vi "DAQ Frequency Meter.vi"() -> ()   [LabVIEW 2013]
doc: "Use this template to build a standard state machine design pattern. Each state executes code and determines which state to transition to. Contrast this design pattern with the User Interface Event Handler pattern, in which code executes in response to user actions. Contrast this design pattern also with the Queued Message Handler pattern, in which each message handling code can queue zero or more new messages.\nNote: This template does not contain the most recent programming guidelines recommended by National Instruments. For a complete, project-based implementation of the Standard State Machine pattern, use the Create Project dialog box instead of this template."
uses:
  DAQ_Count_States.ctl
  <vilib>/DAQmx/read.llb/DAQmx Read (Counter DBL 1Chan 1Samp).vi
  globals_9.vi
  <vilib>/DAQmx/create/channels.llb/DAQmx Create Channel (CI-Period).vi
  <vilib>/DAQmx/create/channels.llb/DAQmx Create Channel (CI-Frequency).vi
  <vilib>/DAQmx/miscellaneous.llb/DAQmx Fill In Error Info.vi
  <resource>/objmgr/daqmx.rc
panel:
  in  "stop":bool
  out "data":dbl caption="Frequency, Hz" format="%_8p"
  in  "mode":enum16{"period", "frequency"}(ring)
  in  "terminal":tag
  in  "counter":tag
  in  "measurement method":i32(ring)=10105 items=["Low Frequency with 1 Counter"=10105, "High Frequency with 2 Counters"=10157, "Large Range with 2 Counters"=10205, "Dynamic Averaging"=16065]
  in  "minimum value":dbl=2.0 format="%0.6f"
  in  "maximum value":dbl=100.0 format="%0.6f"
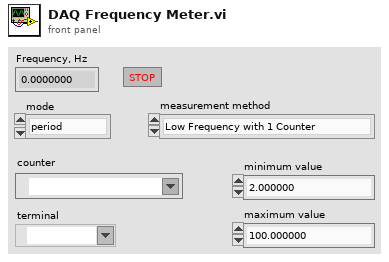
[diagram p1: front panel]
types:
  T1 = typedef "DAQ_Count_States.ctl" = enum16{"Initialize", "Stop", "Read"}
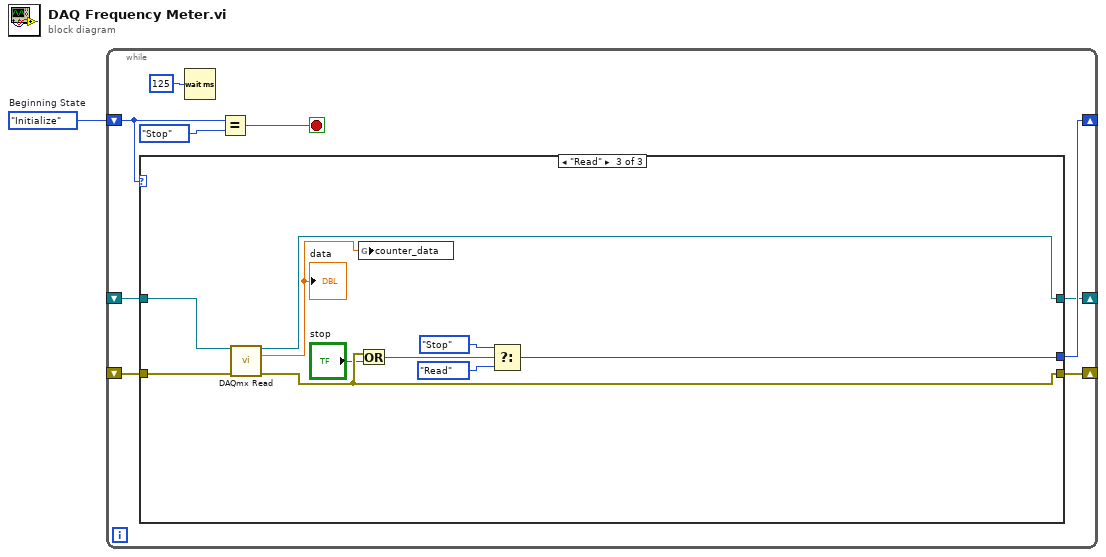
[diagram p0: block diagram]
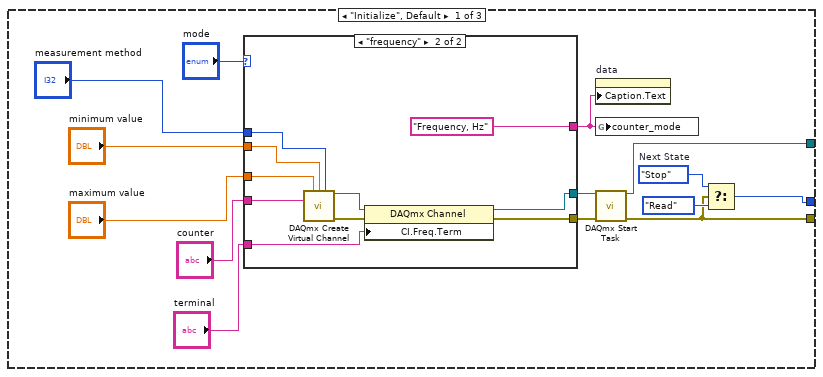
[diagram p2: hidden frame]
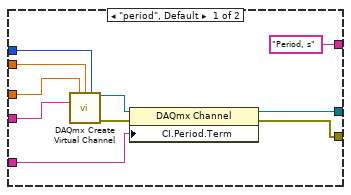
[diagram p3: hidden frame]
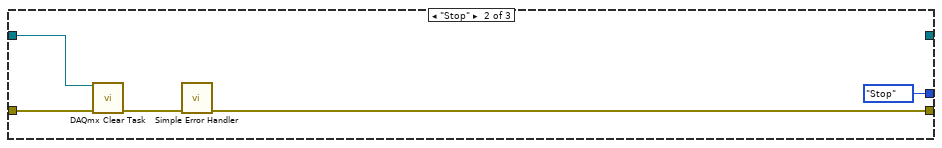
[diagram p4: hidden frame]
diagram:
  w1 = DAQ_Count_States."Initialize"  # Beginning State
  n1 = while {
    shift-right: [w7] -> _
    shift-left: w1 -> [w8]
    shift-right: [w5] -> _
    shift-left: _ -> [w3]
    shift-right: [w4] -> _
    shift-left: _ -> [w2]
    stop <- w10 stop-if-true
    n2 = case shown="\"Read\"" w8 {
      tunnel: [w12 DAQ_Count_States."Stop" ("Next State") w52] -> w7
      tunnel: [w16 _ w58] -> w5
      tunnel: [w14 w48 w56] -> w4
      tunnel: w3 -> [_ w47 w59]
      tunnel: w2 -> [_ w46 w57]
      frame "Initialize", Default {
        w13 = DAQ_Count_States."Stop"  # Next State
        n3 = case shown="\"frequency\"" "mode" {
          tunnel: "terminal" -> [w34 w44]
          tunnel: "counter" -> [w33 w43]
          tunnel: "maximum value" -> [w32 w42]
          tunnel: "minimum value" -> [w31 w41]
          tunnel: "measurement method" -> [w30 w40]
          tunnel: [w27 w37] -> w18
          tunnel: [w26 w36] -> w17
          tunnel: ["Period, s" "Frequency, Hz"] -> w11
          frame "period", Default {
            n4 = call-poly <vilib>:"DAQmx Create Virtual Channel.vi"("maximum value"=w32, "minimum value"=w31, "measurement method"=w30, "counter"=w33) -> ("task out"=w28:refnum<k21>, "error out"=w29:errorcluster)  [unwired: 10 in]
            n5 = property class="DAQmx Channel"(reference=w28, error in=w29, "CI.Period.Term"=w34) -> (reference out=w27:refnum<k21>, error out=w26:errorcluster)
          }
          frame "frequency" {
            n6 = call-poly <vilib>:"DAQmx Create Virtual Channel.vi"("maximum value"=w42, "minimum value"=w41, "measurement method"=w40, "counter"=w43) -> ("task out"=w38:refnum<k21>, "error out"=w39:errorcluster)  [unwired: 10 in]
            n7 = property class="DAQmx Channel"(reference=w38, error in=w39, "CI.Freq.Term"=w44) -> (reference out=w37:refnum<k21>, error out=w36:errorcluster)
          }
        }
        n8 = property on="data" class="DigNum (strict)"("Caption.Text"=w11) -> ()  [unwired: 2 in, 2 out]
        n9 = global write "globals_9.vi" "counter_mode"(w11) -> ()
        n10 = call <vilib>:"DAQmx Start Task.vi"("task/channels in"=w18, "error in"=w17) -> ("task out"=w16:refnum<k21>, "error out"=w14:errorcluster)  [unwired: 12 in]
        n11 = Select(t=w13, s=w14, f=DAQ_Count_States."Read") -> (s? t:f=w12:T1)
      }
      frame "Stop" {
        n12 = call <vilib>:"DAQmx Clear Task.vi"("task in"=w47, "error in"=w46) -> ("error out"=w45:errorcluster)  [unwired: 13 in]
        n13 = call <vilib>:"Simple Error Handler.vi"("error in (no error)"=w45) -> ("error out"=w48:errorcluster)  [unwired: 4 in, 4 out]
      }
      frame "Read" {
        n14 = call-poly <vilib>:"DAQmx Read.vi"("task/channels in"=w59, "error in"=w57) -> ("task out"=w58:refnum<k21>, "data"=w50:dbl, "error out"=w56:errorcluster)  [unwired: 11 in]
        "data" <- w50
        n15 = global write "globals_9.vi" "counter_data"(w50) -> ()
        n16 = Or(x=w56, y="stop") -> (x .or. y?=w55:bool)
        n17 = Select(t=DAQ_Count_States."Stop" ("States"), s=w55, f=DAQ_Count_States."Read" ("States")) -> (s? t:f=w52:T1)
      }
    }
    n18 = Wait (ms)(milliseconds to wait=u32 125) -> ()  [unwired: 1 out]
    n19 = Equal?(x=w8, y=DAQ_Count_States."Stop" ("States")) -> (x = y?=w10:bool)
  }
